vi "Read.vi"(11 "GroupsValue in":refnum<class "GroupsValue.lvclass">) -> (2 "Groups":string[](array[string]))   [LabVIEW 2020, in "Vecto.lvlib" / "GroupsValue.lvclass"]
uses:
  GroupsValue.lvclass
  GroupsValue.lvclass/GroupsValue.ctl
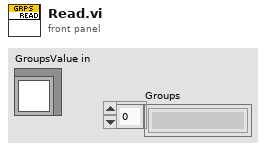
[diagram p1: front panel]
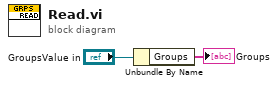
[diagram p0: block diagram]
diagram:
  n1 = Unbundle By Name("GroupsValue in") -> ("Groups"=→"Groups":string[])
